vi "Destroy.vi"(0 "reference in":refnum<class "LcWebView.lvclass">, 5 "Error In":errorcluster) -> (14 "reference out":refnum<class "LcWebView.lvclass">, 19 "Error Out":errorcluster)   [LabVIEW 2019, in "LcWebView.lvclass"]
uses:
  LcWebView.lvclass
  C:/Projects/WebView2/LcWebView/data/Microsoft.Web.WebView2.WinForms.dll
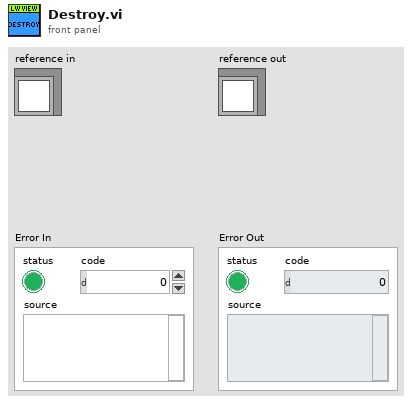
[diagram p1: front panel]
types:
  T1 = typedef "LcWebView.lvclass/ObjectAttributes.ctl" = cluster{"WebView Container":refnum<k24>, "CoreWebViewRef":refnum<k24>, "Status":i32, "Status Message":string, "User Data Folder":path, "DynamicEvents":T2, "BrowserProcessId":u32, "PlotMap":T3, "PlotType":T5}
  T2 = typedef "LcWebView.lvclass/WebViewDynamicEvents.ctl" = cluster{"Event Registration Ref":refnum<event-registration>, "Source event":refnum<user-event>}
  T3 = typedef "LcWebView.lvclass/PlotMap.ctl" = map{string, T4}
  T4 = typedef "LcWebView.lvclass/PlotRef.ctl" = cluster{"PlotType":T5, "PlotTemplate":string}
  T5 = typedef "LcWebView.lvclass/PlotType.ctl" = enum16{"bar", "line", "pie"}
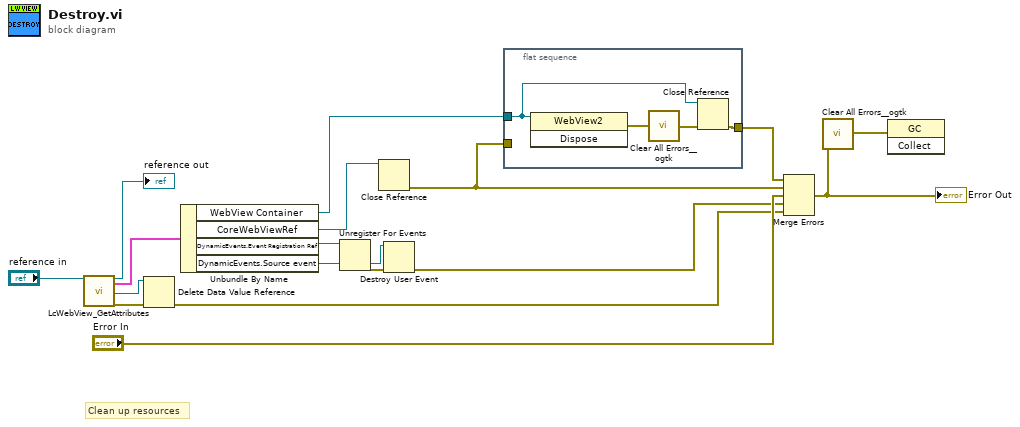
[diagram p0: block diagram]
diagram:
  # "Clean up resources"
  n1 = call "LcWebView_GetAttributes.vi"("reference in"="reference in") -> ("reference out"=→"reference out":refnum<class "LcWebView.lvclass">, "Data"=w13:T1, "DataRef"=w14:refnum<data-value>, "error out"=w15:errorcluster)  [unwired: 15 in]
  n2 = Delete Data Value Reference(data value reference=w14, error in=w15) -> (error out=w5:errorcluster)  [unwired: 1 out]
  n3 = Unbundle By Name(w13) -> ("WebView Container"=w4:refnum<k24>, "CoreWebViewRef"=w11:refnum<k24>, "DynamicEvents.Event Registration Ref"=w9:refnum<event-registration>, "DynamicEvents.Source event"=w7:refnum<user-event>)
  n4 = Unregister For Events(event registration refnum=w9) -> (error out=w8:errorcluster)  [unwired: 1 in]
  n5 = Close Reference(reference=w11) -> (error out=w1:errorcluster)  [unwired: 1 in]
  n6 = Destroy User Event(user event=w7, error in=w8) -> (error out=w6:errorcluster)
  n7 = flat-sequence {
    tunnel: [w21] -> w10
    tunnel: w4 -> [w20]
    tunnel: w1 -> [_]
    frame #0 {
      n8 = invoke class="WebView2" method="Dispose"(reference=w20) -> (error out=w19:errorcluster)  [unwired: 2 in, 2 out]
      n9 = call "Clear All Errors__ogtk.vi"("Error In"=w19) -> ("Error Out"=w18:errorcluster)  [unwired: 3 in]
      n10 = Close Reference(reference=w20, error in (no error)=w18) -> (error out=w21:errorcluster)
    }
  }
  n11 = Merge Errors(w10, w1, "Error In", w6, w5) -> (w3:errorcluster)
  "Error Out" <- w3
  n12 = call "Clear All Errors__ogtk.vi"("Error In"=w3) -> ("Error Out"=w2:errorcluster)  [unwired: 3 in]
  n13 = invoke class="GC" method="Collect"(error in=w2) -> ()  [unwired: 2 in, 3 out]
